vi "ScaleSqWaveParams.vi"(8 "error in (no error)":errorcluster, 9 "clock rate (Hz)":dbl=40000000.0 format="%#_6p", 10 "max voltage for target":dbl=5.0, 11 "square wave props":T2={"frequency (Hz)"=10000.0, "phase offset (deg)"=0.0, "duty cycle (%)"=50.0, "amplitude (V peak)"=10.0, "offset (V)"=0.0} {"frequency (Hz)" format="%#_6p"}) -> (0 "error out":errorcluster, 3 "scaled square wave props":T1 {"frequency (periods/tick)" format="%.32g"; "phase offset (periods)" format="%.32g"; "duty cycle (periods)" format="%.32g"})   [LabVIEW 2021]
uses:
  <vilib>/rvi/Analysis/host/Public/NI_FpgaMspHost.lvlib
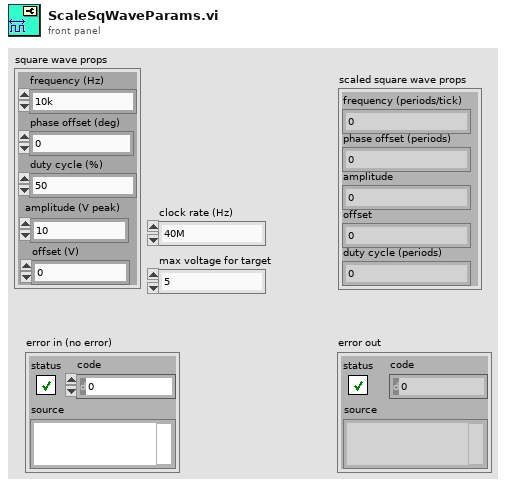
[diagram p1: front panel]
types:
  T1 = cluster{"frequency (periods/tick)":fxp<+,32,0>, "phase offset (periods)":fxp<+,32,0>, "amplitude":i16, "offset":i16, "duty cycle (periods)":fxp<+,32,0>}
  T2 = cluster{"frequency (Hz)":dbl, "phase offset (deg)":dbl, "duty cycle (%)":dbl, "amplitude (V peak)":dbl, "offset (V)":dbl}
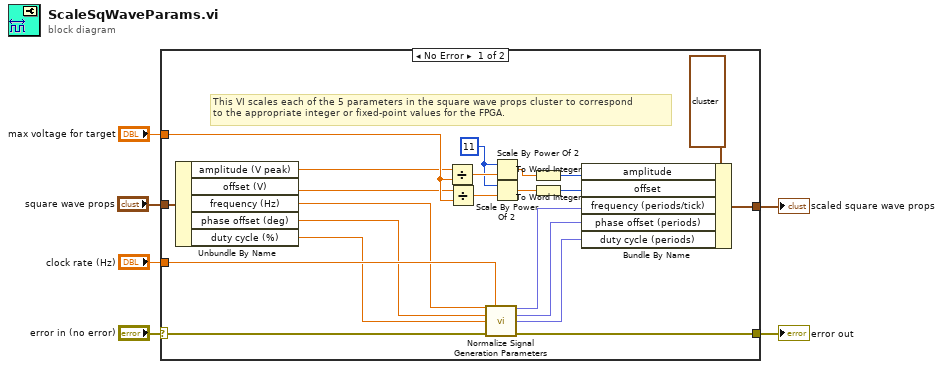
[diagram p0: block diagram]
diagram:
  n1 = case shown="No Error" "error in (no error)" {
    selector: "error in (no error)" -> [w19 w29]
    tunnel: [w28 _] -> w6
    tunnel: "square wave props" -> [w22 _]
    tunnel: "clock rate (Hz)" -> [w18 _]
    tunnel: "max voltage for target" -> [w21 _]
    tunnel: [w15 w29] -> w1
    frame No Error {
      w25 = 11 ("n")
      # "This VI scales each of the 5 parameters in the square wave props cluster to correspond\nto the appropriate integer or fixed-point values for the FPGA."
      n2 = Unbundle By Name(w22) -> ("amplitude (V peak)"=w7:dbl, "offset (V)"=w11:dbl, "frequency (Hz)"=w8:dbl, "phase offset (deg)"=w17:dbl, "duty cycle (%)"=w16:dbl)
      n3 = Divide(x=w7, y=w21) -> (x/y=w27:dbl)
      n4 = Divide(x=w11, y=w21) -> (x/y=w26:dbl)
      n5 = call <vilib>:"Normalize Signal Generation Parameters.vi"("frequency (Hz)"=w8, "FPGA clock rate (Hz)"=w18, "phase offset (deg)"=w17, "duty cycle (%)"=w16, "error in (no error)"=w19) -> ("frequency (periods/tick)"=w14:fxp<+,32,0>, "phase offset (periods)"=w13:fxp<+,32,0>, "duty cycle (periods)"=w12:fxp<+,32,0>, "error out"=w15:errorcluster)  [unwired: 5 in, 2 out]
      n6 = Scale By Power Of 2(n=w25, x=w27) -> (x*2^n=w24:dbl)
      n7 = Scale By Power Of 2(n=w25, x=w26) -> (x*2^n=w23:dbl)
      n8 = To Word Integer(number=w24) -> (16bit integer=w10:i16)
      n9 = To Word Integer(number=w23) -> (16bit integer=w9:i16)
      n10 = Bundle By Name(cluster=T1 {"frequency (periods/tick)"=0.9999999997671694, "phase offset (periods)"=0.0, "amplitude"=4096, "offset"=0, "duty cycle (periods)"=0.9999999997671694} ("Square wave 3"), "amplitude"=w10, "offset"=w9, "frequency (periods/tick)"=w14, "phase offset (periods)"=w13, "duty cycle (periods)"=w12) -> (w28:T1)
    }
    frame Error {
    }
  }
  "scaled square wave props" <- w6
  "error out" <- w1
